vi "PhaSER-2C.vi"() -> ()   [LabVIEW 2017]
uses:
  Analog_Channels.ctl
  state_enum.ctl
  <vilib>/Analysis/3filter.llb/Filter Passband Type.ctl
  <vilib>/Analysis/3filter.llb/Filter Structure Type.ctl
  <vilib>/Utility/error.llb/DialogType.ctl
  <vilib>/DAQmx/read.llb/DAQmx Read (Analog 1D Wfm NChan NSamp).vi
  <vilib>/DAQmx/write.llb/DAQmx Write (Digital Bool 1Line 1Point).vi
  <vilib>/DAQmx/miscellaneous.llb/DAQmx Fill In Error Info.vi
  <vilib>/Analysis/3filter.llb/Zero Phase Filter (DBL).vi
  <vilib>/DAQmx/create/channels.llb/DAQmx Create Channel (AI-Voltage-Basic).vi
  <vilib>/DAQmx/configure/timing.llb/DAQmx Timing (Sample Clock).vi
  <vilib>/DAQmx/create/channels.llb/DAQmx Create Channel (DO-Digital Output).vi
  <vilib>/DAQmx/create/channels.llb/DAQmx Create Channel (CO-Pulse Generation-Time).vi
  <resource>/objmgr/daqmx.rc
  <vilib>/Analysis/NI_AALBase.lvlib
  <vilib>/ptbypt/NI_PtbyPt.lvlib
panel:
  in  "zero phase order":i32=1
  in  "low cutoff":dbl=4.0 format="%0.3f"
  in  "high cutoff":dbl=9.0 format="%0.3f"
  in  "Inhibition End":dbl=-45.0
  in  "Inhibtion Start":dbl=45.0
  in  "Inhibition Channel":tag="Dev1/PFI13"
  in  "timeout":dbl=100.0 caption="Pulse Timeout (ms)"
  in  "pulse phase":dbl format="%#_13g"
  in  "Counter":tag="Dev1/ctr0"
  in  "Output Terminal":tag="/Dev1/PFI12"
  in  "Pulse Duration":dbl=0.001 format="%.6f"
  out "Ball Tracker":i32=3
  out "Inhibition":i32=-1
  out "Pulse Train":i32=2
  out "Trigger":i32=1
  out "LFP":i32
  in  "Channel Assignments":T1[](array[typedef])=[enum."LFP", enum."Trigger", enum."Pulse Train", enum."Ball Tracker", enum."Inhibition"]
  in  "Samples to read":i32=25
  in  "Sample Rate":dbl=25000.0
  in  "Max Voltage":dbl=2.0
  in  "Min Voltage":dbl=-1.0
  in  "Physical Channel":tag="Dev1/ai0:4"
  in  "restrict to running?":bool=TRUE
  in  "fractional run threshold":dbl=0.1
  in  "lower speed bound":dbl=2.4 format="%#_13g"
  in  "upper speed bound":dbl=2.7 format="%#_13g"
  in  "sample length (ms)":i32=1000
  in  "Base Filename":path=path "C:/Users/Paul/Desktop/LabVIEW_Recordings/test"
  in  "Quit Button":bool
  in  "Stop Button":bool
  in  "Stimulate Button":bool
  in  "Baseline Button":bool
  in  "thickness":i32=150
  in  "width":i32=1000
  in  "p":dbl=13.0
  out "Waveform Chart":waveform(dbl)[](graph)=[{"t0"=timestamp(3702733252.213229 s since 1904-01-01), "dt"=0.001, "Y"=[-0.49778657094501827], "attributes"=variant("NI_ChannelName"=variant(string "Silicon Probe"), "NI_UnitDescription"=variant(string "Volts"))}, {"t0"=timestamp(3702733252.2132373 s since 1904-01-01), "dt"=3.9999999999999996e-05, "Y"=[0.0012770261409516398, 0.0009479371254728086, 0.0007833926177167883, 0.0009479371254728086, 0.0011124816332177545, 0.0009479371254728086, 0.0011124816332177545, 0.0009479371254728086, 0.0011124816332177545, 0.0009479371254728086, 0.0007833926177167883, 0.0007833926177167883, 0.0011124816332177545, 0.0011124816332177545, 0.0007833926177167883, 0.0011124816332177545, 0.0011124816332177545, 0.0007833926177167883, 0.0009479371254728086, 0.0009479371254728086, 0.0007833926177167883, 0.0011124816332177545, 0.0007833926177167883, 0.0011124816332177545, 0.0011124816332177545], "attributes"=variant("NI_ChannelName"=variant(string "Trigger"), "NI_UnitDescription"=variant(string "Volts"))}, {"t0"=timestamp(3702733252.2132454 s since 1904-01-01), "dt"=3.9999999999999996e-05, "Y"=[0.004897005308322218, 0.0045679162933244324, 0.004897005308322218, 0.0045679162933244324, 0.004732460800828724, 0.0045679162933244324, 0.004732460800828724, 0.004403371785809317, 0.004732460800828724, 0.0045679162933244324, 0.004732460800828724, 0.0045679162933244324, 0.004403371785809317, 0.004732460800828724, 0.004732460800828724, 0.0045679162933244324, 0.004403371785809317, 0.004732460800828724, 0.004732460800828724, 0.004403371785809317, 0.004732460800828724, 0.004732460800828724, 0.004403371785809317, 0.0045679162933244324, 0.005390638830738002], "attributes"=variant("NI_ChannelName"=variant(string "Pulse Train"), "NI_UnitDescription"=variant(string "Volts"))}, {"t0"=timestamp(3702733252.213253 s since 1904-01-01), "dt"=3.9999999999999996e-05, "Y"=[2.6063520142436025, 2.603883827309811, 2.6040483731041806, 2.608162018019915, 2.60668110583773, 2.5999347282970344, 2.604212918898724, 2.6052001936696327, 2.6117820256357307, 2.607174743230226, 2.607503834826093, 2.609972021817286, 2.6010865488321, 2.607174743230226, 2.5948338088867064, 2.602402915168302, 2.605858376853715, 2.604212918898724, 2.5890747065265556, 2.609478384415914, 2.607503834826093, 2.6043774646934414, 2.6027320067540884, 2.6043774646934414, 2.604542010488332], "attributes"=variant("NI_ChannelName"=variant(string "Ball Tracker"), "NI_UnitDescription"=variant(string "Volts"))}, {"t0"=timestamp(3702733252.213261 s since 1904-01-01), "dt"=3.9999999999999996e-05, "Y"=[2.562418292635671, 2.561924655383818, 2.5632410213921757, 2.5632410213921757, 2.5632410213921757, 2.563899204400454, 2.5637346586481278, 2.5637346586481278, 2.564063750152951, 2.5637346586481278, 2.563570112895973, 2.5625828383866303, 2.561760109633542, 2.562089201134265, 2.561266472383738, 2.562089201134265, 2.5622537468848825, 2.562089201134265, 2.562089201134265, 2.5622537468848825, 2.5622537468848825, 2.562418292635671, 2.562418292635671, 2.562089201134265, 2.5634055671439886], "attributes"=variant("NI_ChannelName"=variant(string "Inhibition"), "NI_UnitDescription"=variant(string "Volts"))}, {"t0"=timestamp(3702733252.213229 s since 1904-01-01), "dt"=0.001, "Y"=[0.32829558433683736], "attributes"=variant("NI_ChannelName"=variant(string "Predicted Signal"), "NI_UnitDescription"=variant(string "Volts"))}]
  out "Status":string="Quitting Program"
  # "Filter Parameters"
  # "Excitation Trigger"
  # "Inhibition TTL"
  # "Analog In Channels"
  # "Channel Number:"
  # "Analog In 0"
  # "Analog In 1"
  # "Analog In 2"
  # "Analog In 3"
  # "Analog In 4"
  # "Ball Tracker Parameters"
  # "Autoregression Parameters"
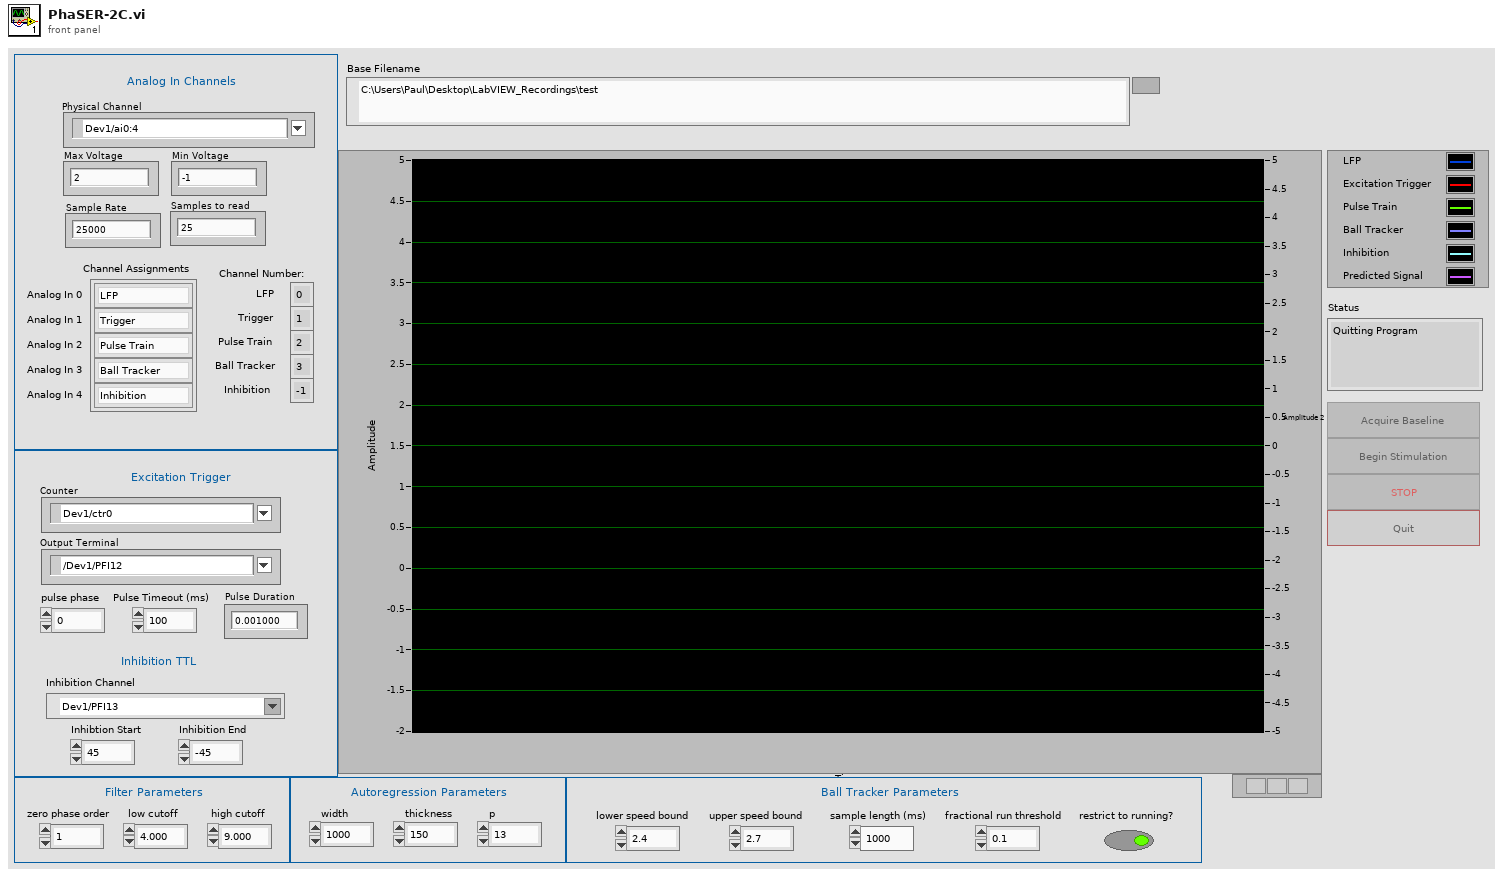
[diagram p1: front panel]
types:
  T1 = typedef "Analog_Channels.ctl" = enum16{"LFP", "Trigger", "Pulse Train", "Glass Electrode", "Ball Tracker", "Inhibition"}
  T2 = typedef "DialogType.ctl" = u16
  T3 = typedef "NI_AALBase.lvlib/Filter Structure Type.ctl" = u16
  T4 = typedef "NI_AALBase.lvlib/Filter Passband Type.ctl" = enum32{"Lowpass", "Highpass", "Bandpass", "Bandstop"}
  T5 = typedef "state_enum.ctl" = enum16{"Wait", "Locate", "Stop", "Quit", "Baseline", "Artifact", "Stimulate", "Initialize"}
  T6 = cluster{"filter structure":enum32{"IIR 2nd Order", "IIR 4th Order"}, "Reverse Coefficients":dbl[], "Forward Coefficients":dbl[]}
  T7 = enum16{"open", "open or create", "create or replace", "create", "open (read-only)"}
  T8 = enum8{"Enabled", "Disabled", "Disabled and Grayed Out"}
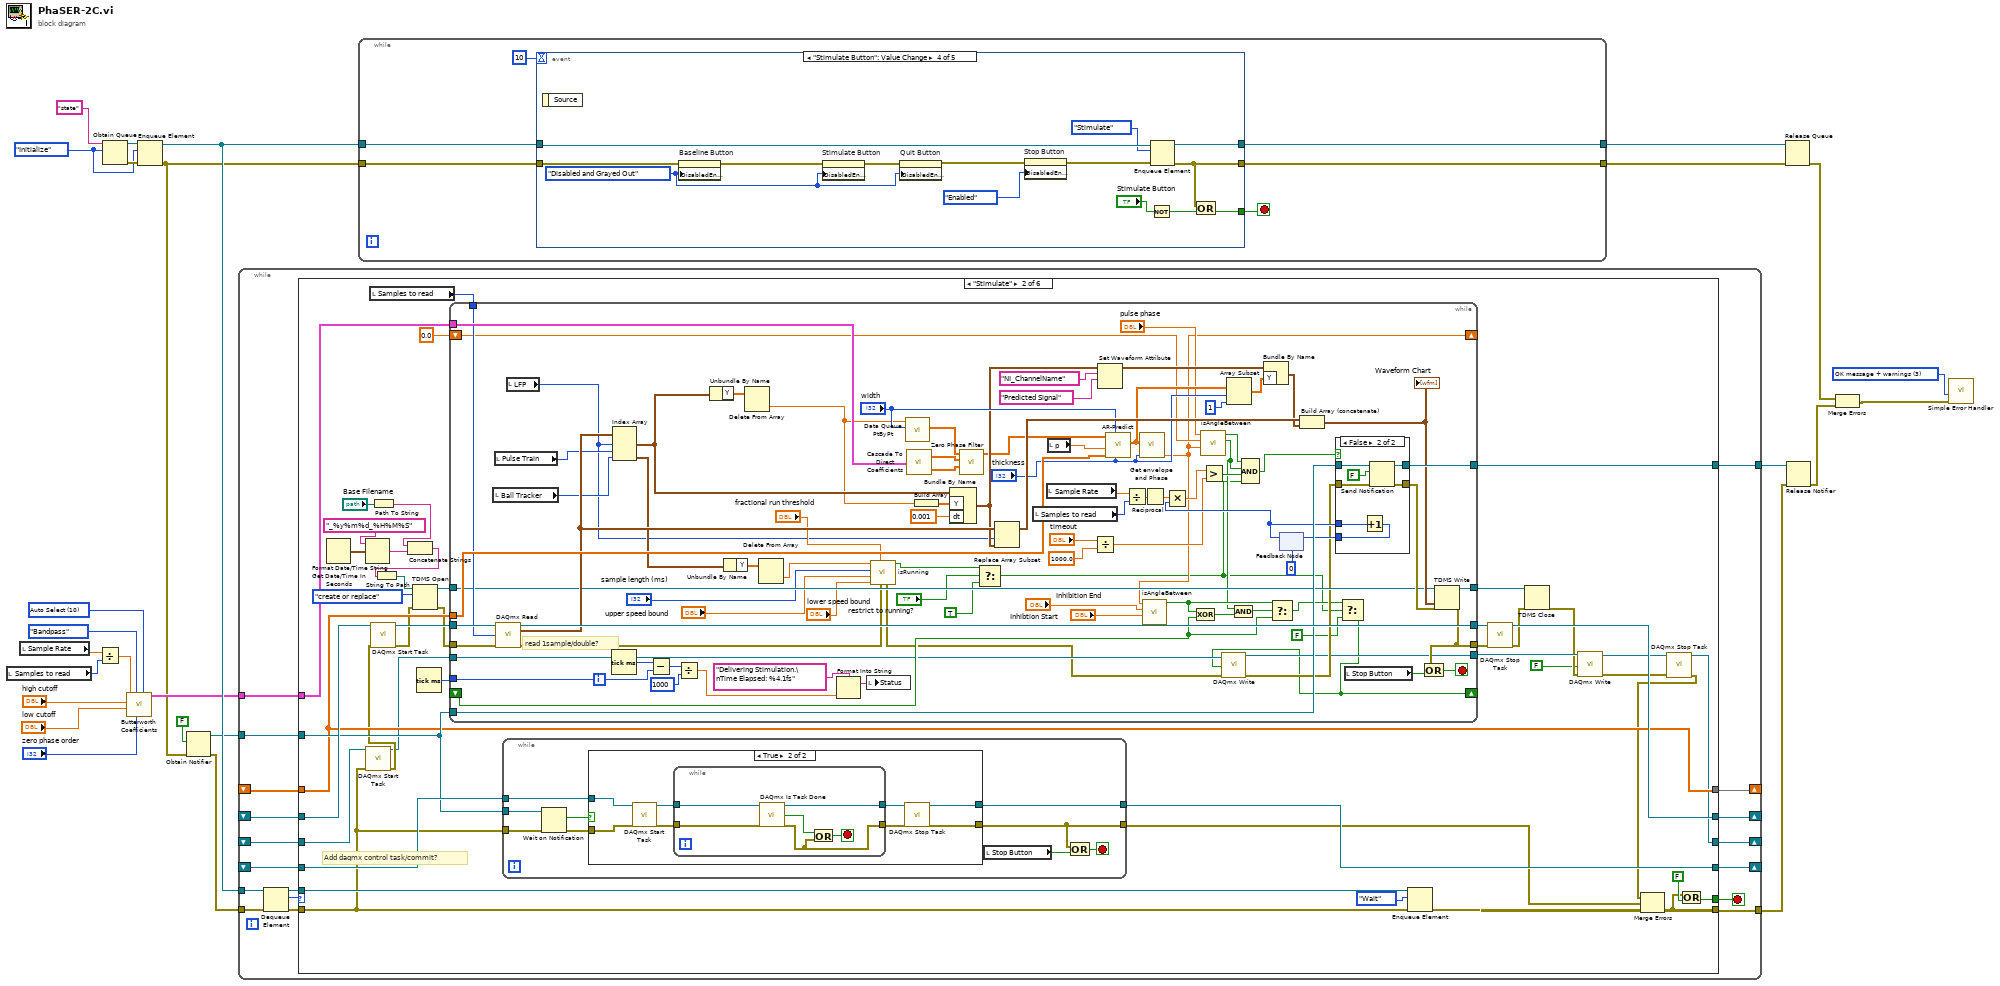
[diagram p0: block diagram]
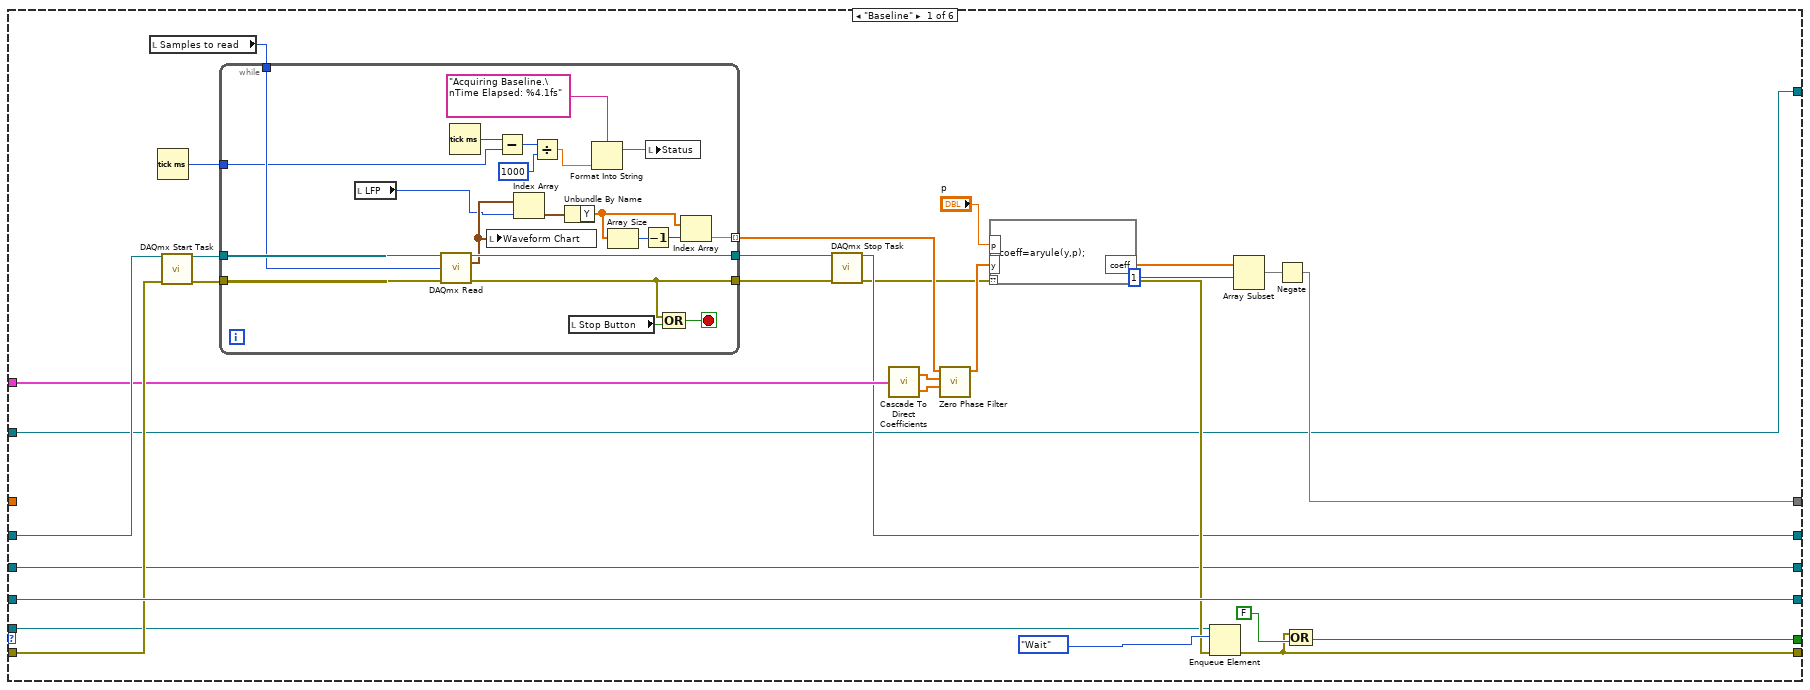
[diagram p2: hidden frame]
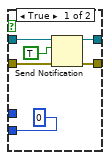
[diagram p4: hidden frame]
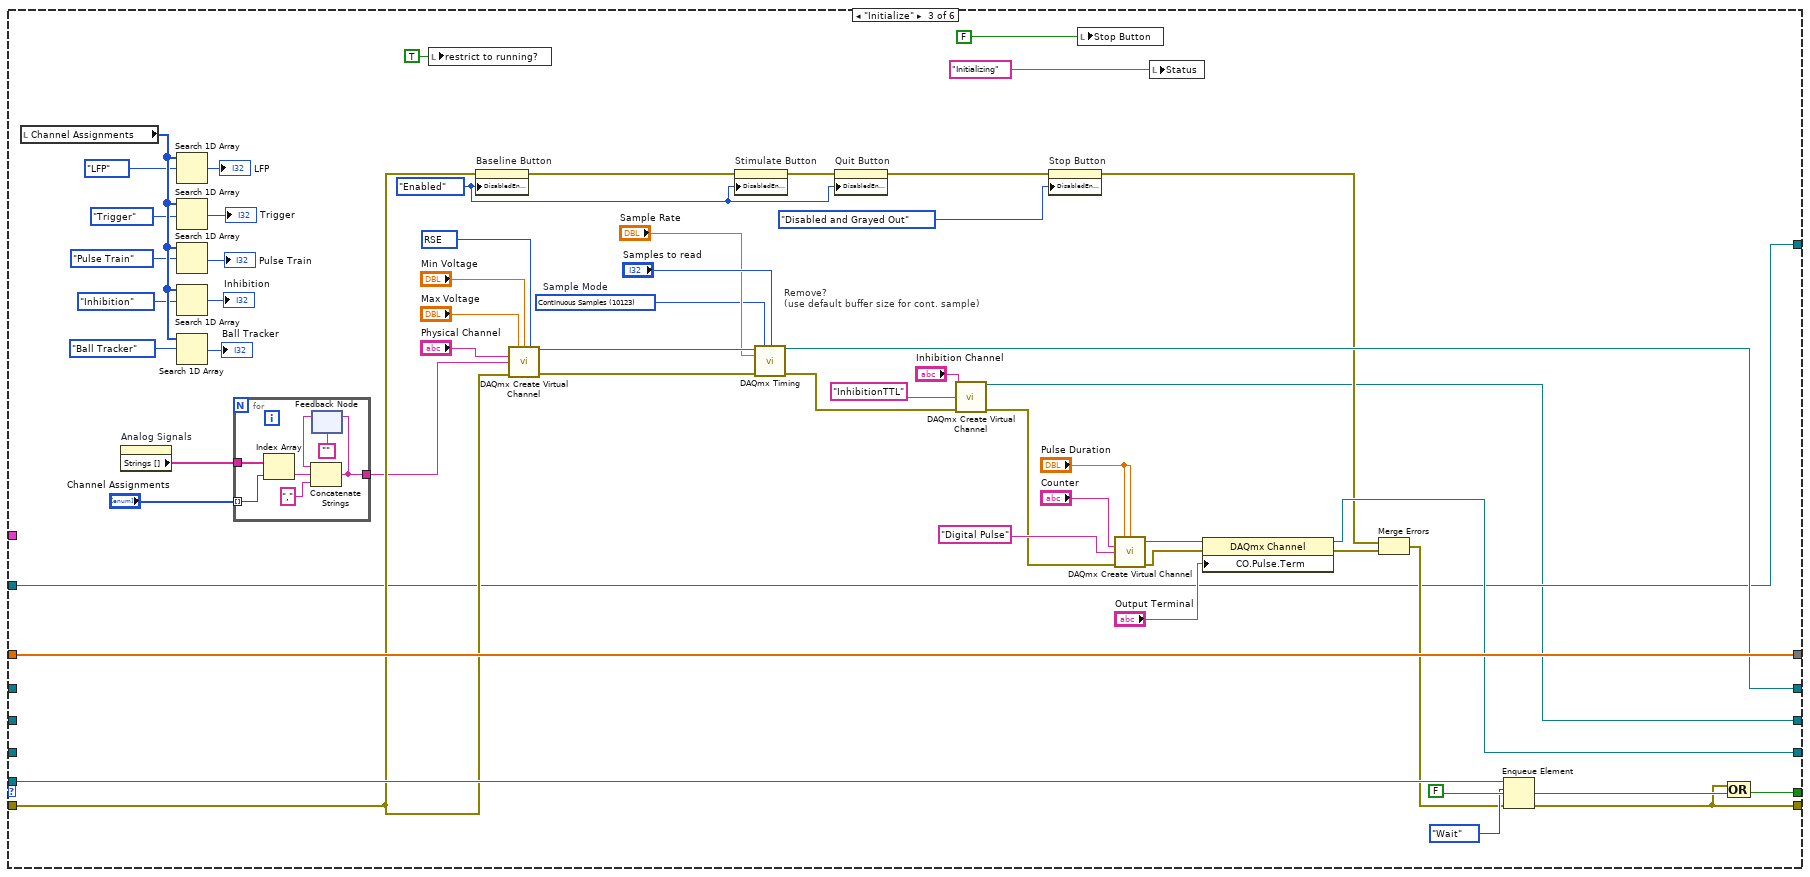
[diagram p5: hidden frame]
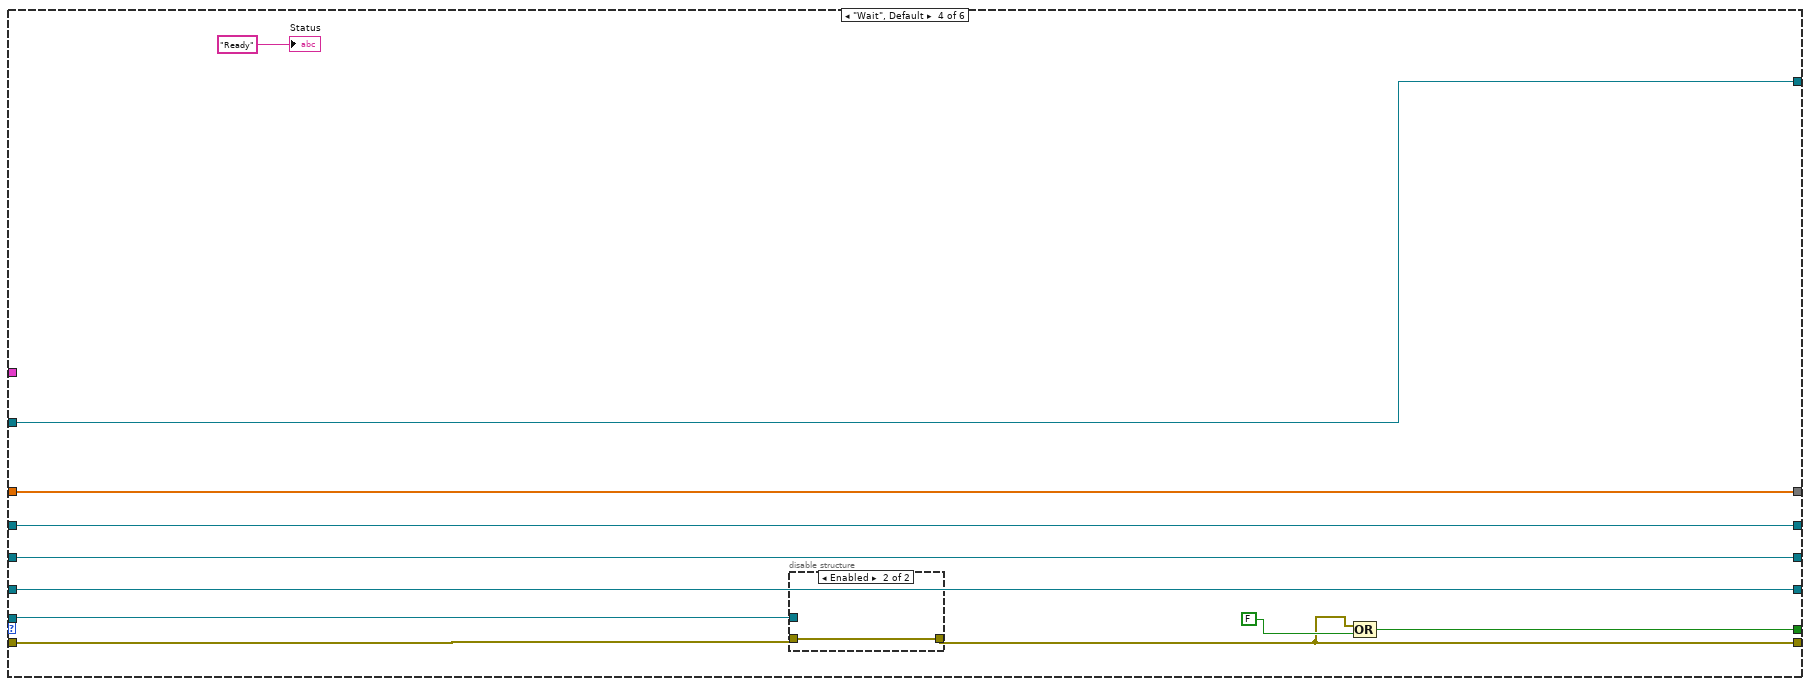
[diagram p6: hidden frame]
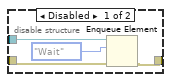
[diagram p7: hidden frame]
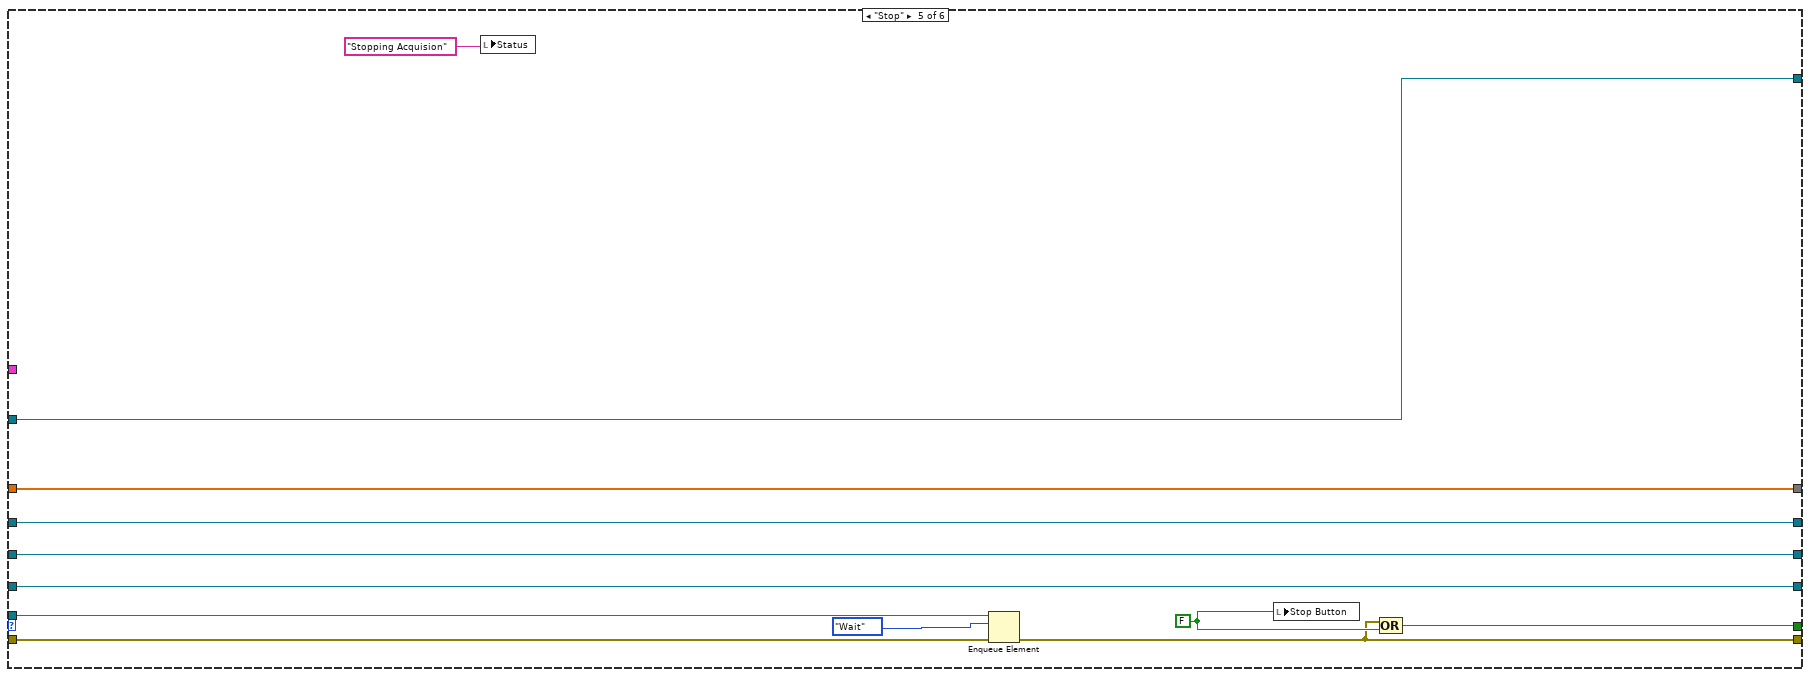
[diagram p8: hidden frame]
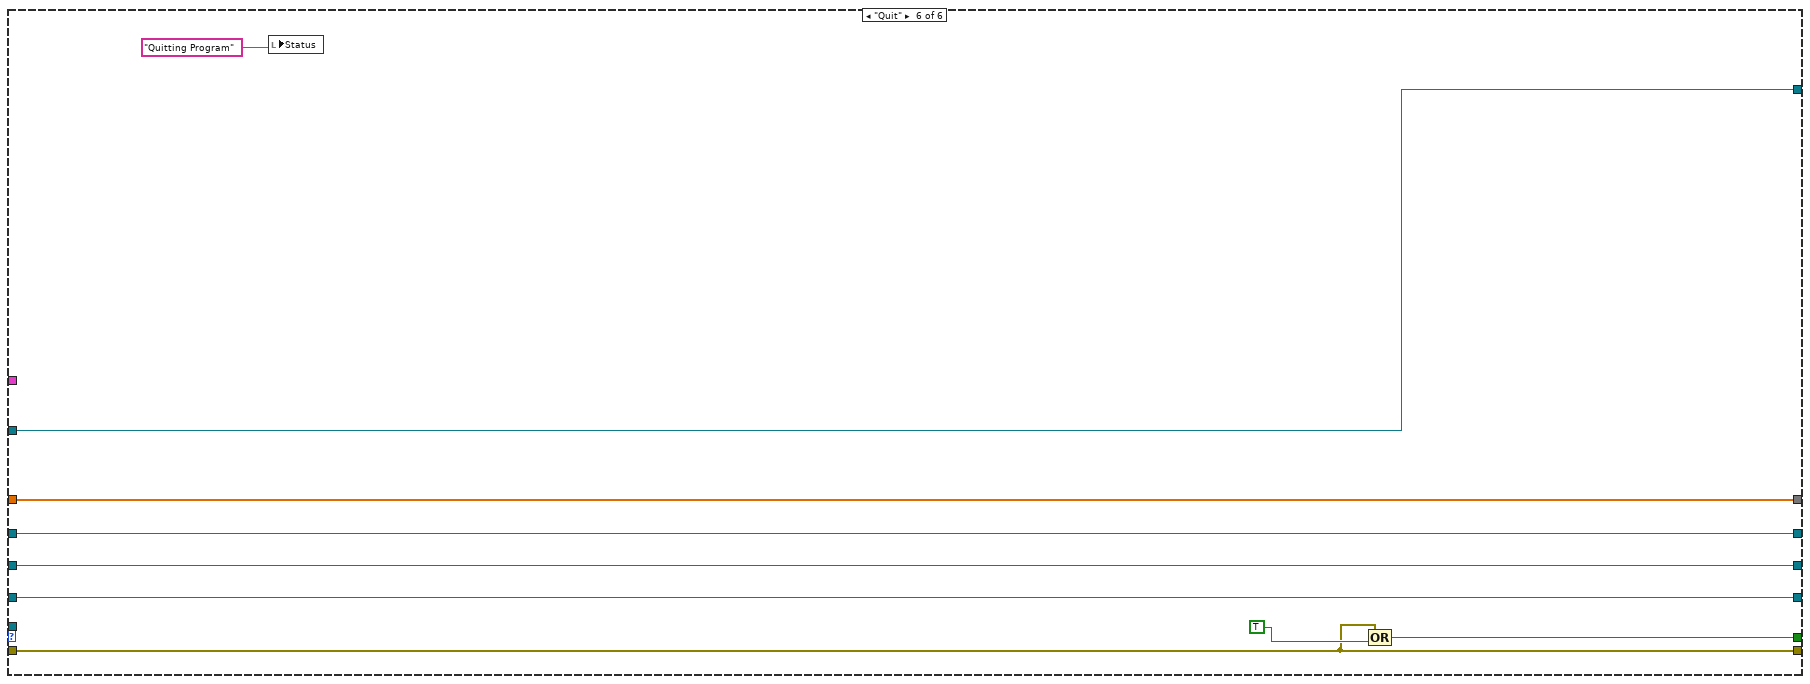
[diagram p9: hidden frame]
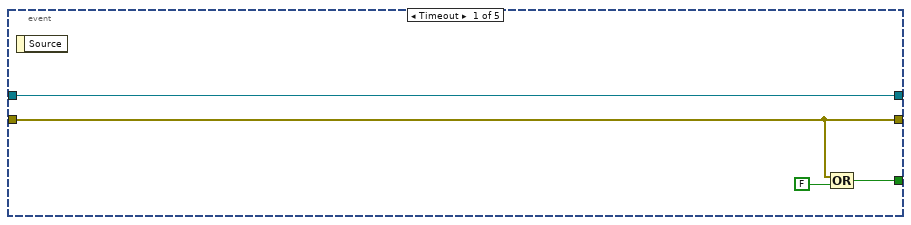
[diagram p10: hidden frame]
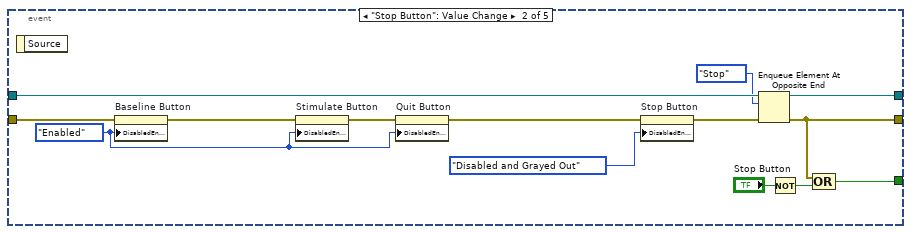
[diagram p11: hidden frame]
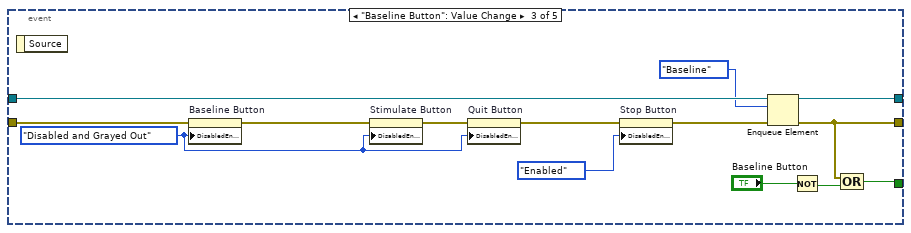
[diagram p12: hidden frame]
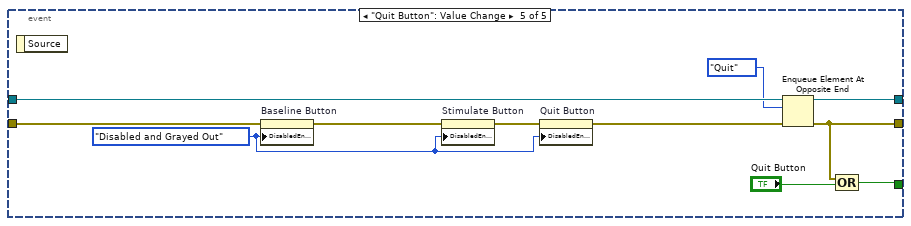
[diagram p13: hidden frame]
diagram:
  w9 = T2 3 items=["no dialog", "OK message", "continue or stop message", "OK message + warnings", "continue/stop + warnings"] ("type of dialog (OK msg:1)")
  w17 = T3 10 items=["IIR 2nd Order"=0, "IIR 4th Order"=1, "Auto Select"=10] ("filter structure option")
  w23 = state_enum."Initialize"
  n1 = local read "Samples to read"() -> (w4:i32)
  n2 = local read "Sample Rate"() -> (w14:dbl)
  n3 = Divide(x=w14, y=w4) -> (x/y=w1:dbl)
  n4 = Obtain Queue(name (unnamed)="state", element data type=w23) -> (queue out=w25:refnum<queue>, error out=w24:errorcluster)  [unwired: 3 in, 1 out]
  n5 = call <vilib>:"Butterworth Coefficients.vi"("filter structure option"=w17, "order"="zero phase order", "filter type"=Filter_Passband_Type."Bandpass", "low cutoff freq: fl"="low cutoff", "high cutoff freq: fh"="high cutoff", "sampling freq: fs"=w1) -> ("IIR Filter Cluster"=w15:T6)  [unwired: 4 in, 1 out]
  n6 = Enqueue Element(queue=w25, element=w23, error in (no error)=w24) -> (queue out=w22:refnum<queue>, error out=w11:errorcluster)  [unwired: 1 in, 1 out]
  n7 = Obtain Notifier(notification data type=FALSE, error in (no error)=w11) -> (notifier out=w12:refnum<notifier>, error out=w10:errorcluster)  [unwired: 1 in, 2 out]
  n8 = while {
    tunnel: w22 -> [w44]
    tunnel: [w41] -> w6
    shift-right: [w39] -> _
    shift-left: _ -> [w37]
    shift-right: [w38] -> _
    shift-left: _ -> [w36]
    tunnel: w15 -> [w34]
    shift-right: [w33] -> _
    shift-left: _ -> [w32]
    tunnel: w12 -> [w31]
    tunnel: w10 -> [w30]
    tunnel: [w29] -> w7
    shift-right: [w28] -> _
    shift-left: _ -> [w27]
    stop <- w40 stop-if-true
    n9 = Dequeue Element(queue=w44, error in (no error)=w30) -> (queue out=w35:refnum<queue>, element=w43:T5, error out=w42:errorcluster)  [unwired: 1 in, 1 out]
    n10 = case shown="\"Stimulate\"" w43 {
      tunnel: [w55 w121 w298 w331 w348 w364] -> w41
      tunnel: w42 -> [w69 w105 w295 w333 w352 w364]
      tunnel: [w72 w138 w321 w339 w349 w365] -> w40
      tunnel: [w49 w129 w300 w338 w357 w363] -> w39
      tunnel: [w71 w123 w301 w337 w356 w362] -> w38
      tunnel: w37 -> [w70 w137 _ w338 w357 w363]
      tunnel: w36 -> [w71 w125 _ w337 w356 w362]
      tunnel: w35 -> [w53 w133 w319 w332 w351 _]
      tunnel: w34 -> [w64 w127 _ _ _ _]
      tunnel: [w57 w122 w318 w336 w355 w361] -> w33
      tunnel: w32 -> [_ w122 w318 w336 w355 w361]
      tunnel: w31 -> [w46 w124 w291 w334 w347 w359]
      tunnel: [w46 w119 w291 w334 w347 w359] -> w29
      tunnel: [w45 w100 w272 w330 w346 w358] -> w28
      tunnel: w27 -> [w45 w104 _ w330 w346 w358]
      frame "Baseline" {
        n11 = local read "Samples to read"() -> (w52:i32)
        n12 = Tick Count (ms)() -> (millisecond timer value=w47:u32)
        n13 = call <vilib>:"DAQmx Start Task.vi"("task/channels in"=w70, "error in"=w69) -> ("task out"=w68:refnum<k21>, "error out"=w67:errorcluster)  [unwired: 12 in]
        n14 = while {
          tunnel: [w88] -> w63 mode=indexing
          tunnel: w68 -> [w87]
          tunnel: w67 -> [w86]
          tunnel: [w85] -> w50
          tunnel: [w84] -> w51
          tunnel: w52 -> [w83]
          tunnel: w47 -> [w81]
          stop <- w93 stop-if-true
          n15 = local read "LFP"() -> (w74:i32)
          n16 = call-poly <vilib>:"DAQmx Read.vi"("task/channels in"=w87, "number of samples per channel"=w83, "error in"=w86) -> ("task out"=w85:refnum<k21>, "data"=w75:waveform(dbl)[], "error out"=w84:errorcluster)  [unwired: 10 in]
          n17 = Tick Count (ms)() -> (millisecond timer value=w82:u32)
          n18 = local write "Waveform Chart"(w75) -> ()
          n19 = Subtract(x=w82, y=w81) -> (x-y=w80:u32)
          n20 = Index Array(array=w75, index=w74) -> (element=w92:waveform(dbl))
          n21 = Divide(x=w80, y=u32 1000) -> (x/y=w78:dbl)
          n22 = Unbundle By Name(w92) -> ("Y"=w89:dbl[])
          n23 = local read "Stop Button"() -> (w94:bool)
          n24 = Format Into String(format string="Acquiring Baseline.\nTime Elapsed: %4.1fs", w78) -> (resulting string=w76:string)  [unwired: 2 in, 1 out]
          n25 = Array Size(array=w89) -> (size(s)=w91:i32)
          n26 = Decrement(x=w91) -> (x-1=w90:i32)
          n27 = local write "Status"(w76) -> ()
          n28 = Compound Arithmetic op=OR(w84, w94) -> (w93:bool)
          n29 = Index Array(array=w89, index=w90) -> (element=w88:dbl)
        }
        n30 = call <vilib>:"DAQmx Stop Task.vi"("task/channels in"=w50, "error in"=w51) -> ("task out"=w49:refnum<k21>, "error out"=w48:errorcluster)  [unwired: 12 in]
        n31 = call <vilib>:"Cascade To Direct Coefficients.vi"("IIR Filter Cluster"=w64) -> ("Reverse Coefficients"=w65:dbl[], "Forward Coefficients"=w66:dbl[])
        n32 = call-poly <vilib>:"Zero Phase Filter.vi"("Forward Coefficients"=w66, "Reverse Coefficients"=w65, "X"=w63) -> ("Filtered X"=w62:dbl[])  [unwired: 7 in, 1 out]
        n33 = script code="coeff=aryule(y,p);"("??"=w48, "p"="p", "y"=w62) -> ("??"=w54:errorcluster, "coeff"=w58:dbl[])
        n34 = Enqueue Element(queue=w53, element=state_enum."Wait", error in (no error)=w54) -> (error out=w55:errorcluster)  [unwired: 1 in, 2 out]
        n35 = Array Subset(array=w58, index=1) -> (w60:dbl[])  [unwired: 1 in]
        n36 = Negate(x=w60) -> (-x=w57:dbl[])
        n37 = Compound Arithmetic op=OR(w55, FALSE) -> (w72:bool)
      }
      frame "Stimulate" {
        # "Add daqmx control task/commit?"
        n38 = Get Date/Time In Seconds() -> (seconds since 1Jan1904=w112:timestamp)
        n39 = Format Date/Time String(time format string (%c)="_%y%m%d_%H%M%S", seconds (now)=w112) -> (date/time string=w109:string)  [unwired: 1 in]
        n40 = call <vilib>:"DAQmx Start Task.vi"("task/channels in"=w104, "error in"=w105) -> ("task out"=w102:refnum<k21>, "error out"=w103:errorcluster)  [unwired: 12 in]
        n41 = local read "Samples to read"() -> (w132:i32)
        n42 = call <vilib>:"DAQmx Start Task.vi"("task/channels in"=w137, "error in"=w103) -> ("task out"=w136:refnum<k21>, "error out"=w117:errorcluster)  [unwired: 12 in]
        n43 = Path To String(path="Base Filename") -> (string=w108:string)
        n44 = Concatenate Strings(w108, w109) -> (w106:string)
        n45 = String To Path(string=w106) -> (path=w107:path)
        n46 = TDMS Open(8:w117, 10:T7."create or replace" ("operation (0:open)"), 11:w107) -> (0:w116:errorcluster, 3:w115:refnum<k34>)  [unwired: 4 in]
        n47 = Tick Count (ms)() -> (millisecond timer value=w128:u32)
        n48 = while {
          tunnel: w136 -> [w252]
          tunnel: w116 -> [w251]
          tunnel: [w250] -> w130
          tunnel: [w199] -> w131
          tunnel: w132 -> [w226]
          tunnel: w128 -> [w249]
          tunnel: w127 -> [w240]
          tunnel: w122 -> [w235]
          shift-right: [w176] -> _
          shift-left: 0.0 -> [w184]
          tunnel: w124 -> [w238]
          tunnel: [w237] -> w119
          tunnel: w115 -> [w200]
          tunnel: [w198] -> w114
          tunnel: w102 -> [w174]
          shift-right: [w167] -> _
          shift-left: _ -> [w175]
          tunnel: [w171] -> w99
          stop <- w253 stop-if-true
          # "read 1sample/double?"
          n49 = local read "Ball Tracker"() -> (w197:i32)
          n50 = local read "Pulse Train"() -> (w206:i32)
          n51 = call-poly <vilib>:"DAQmx Read.vi"("task/channels in"=w252, "number of samples per channel"=w226, "error in"=w251) -> ("task out"=w250:refnum<k21>, "data"=w232:waveform(dbl)[], "error out"=w190:errorcluster)  [unwired: 10 in]
          n52 = local read "LFP"() -> (w166:i32)
          n53 = Tick Count (ms)() -> (millisecond timer value=w234:u32)
          n54 = Index Array(array=w232, index #1=w166, index #2=w206, index #3=w197) -> (element #1=w233:waveform(dbl), element #3=w195:waveform(dbl))  [unwired: 1 out]
          n55 = Subtract(x=w234, y=w249) -> (x-y=w248:u32)
          n56 = Divide(x=w248, y=u32 1000) -> (x/y=w246:dbl)
          n57 = Unbundle By Name(w233) -> ("Y"=w165:dbl[])
          n58 = Unbundle By Name(w195) -> ("Y"=w196:dbl[])
          n59 = Delete From Array(array=w165) -> (deleted portion=w219:dbl)  [unwired: 2 in, 1 out]
          n60 = Delete From Array(array=w196) -> (deleted portion=w194:dbl)  [unwired: 2 in, 1 out]
          n61 = Format Into String(format string="Delivering Stimulation.\nTime Elapsed: %4.1fs", w246) -> (resulting string=w244:string)  [unwired: 2 in, 1 out]
          n62 = local write "Status"(w244) -> ()
          n63 = call "isRunning.vi"("error in (no error)"=w190, "fractional run \nthreshold"="fractional run threshold", "lower\nspeed bound"="lower speed bound", "upper\nspeed bound"="upper speed bound", "sample\nlength (ms)"="sample length (ms)", "ballspeed"=w194) -> ("isRunning?"=w188:bool, "error out"=w173:errorcluster)  [unwired: 4 in]
          n64 = call <vilib>:"Data Queue PtByPt.vi"("sample length"="width", "input data point"=w219) -> ("Current Queue"=w241:dbl[])  [unwired: 5 in, 4 out]
          n65 = call <vilib>:"Cascade To Direct Coefficients.vi"("IIR Filter Cluster"=w240) -> ("Reverse Coefficients"=w243:dbl[], "Forward Coefficients"=w242:dbl[])
          n66 = Build Array(w219) -> (w220:dbl[])
          n67 = Bundle By Name(cluster=w233, "Y"=w220, "dt"=0.001) -> (w228:waveform(dbl))
          n68 = call-poly <vilib>:"Zero Phase Filter.vi"("Forward Coefficients"=w242, "Reverse Coefficients"=w243, "X"=w241) -> ("Filtered X"=w224:dbl[])  [unwired: 7 in, 1 out]
          n69 = Select(t=w188, s="restrict to running?", f=TRUE) -> (s? t:f=w168:bool)
          n70 = Replace Array Subset(array=w232, new element=w228, index=w166) -> (w231:waveform(dbl)[])
          n71 = local read "Samples to read"() -> (w213:i32)
          n72 = local read "Sample Rate"() -> (w212:dbl)
          n73 = local read "p"() -> (w236:dbl)
          n74 = Divide(x="timeout", y=1000.0) -> (x/y=w207:dbl)
          n75 = Set Waveform Attribute(5:"Predicted Signal", 6:"NI_ChannelName", 7:w228) -> (3:w205:waveform(dbl))  [unwired: 1 in, 2 out]
          n76 = call "AR-Predict.vi"("thickness"="thickness", "width"="width", "AR coeff"=w235, "p"=w236, "filtered signal"=w224) -> ("predicted signal"=w223:dbl[])  [unwired: 6 in]
          n77 = Divide(x=w212, y=w213) -> (x/y=w211:dbl)
          n78 = call "Get envelope and Phase.vi"("thickness"="thickness", "signal"=w223) -> ("phase"=w176:dbl)  [unwired: 8 in, 1 out]
          n79 = call "isAngleBetween.vi"("End"="Inhibition End", "Start"="Inhibtion Start", "Angle"=w176) -> ("Between?"=w180:bool)  [unwired: 7 in, 1 out]
          n80 = Reciprocal(x=w211) -> (1/x=w210:dbl)
          n81 = Exclusive Or(1:w175, 2:w180) -> (0:w179:bool)
          n82 = call "isAngleBetween.vi"("End"=w176, "Start"=w184, "Angle"="pulse phase") -> ("Clockwise?"=w177:bool, "Between?"=w183:bool)  [unwired: 7 in]
          n83 = Array Subset(array=w223, index="thickness", length=1) -> (w229:dbl[])
          n84 = And(x=w177, y=w179) -> (x .and. y?=w178:bool)
          n85 = Bundle By Name(cluster=w205, "Y"=w229) -> (w227:waveform(dbl))
          n86 = Select(t=w180, s=w178, f=w175) -> (s? t:f=w170:bool)
          n87 = feedback #1(0) -> (w214:i32)
          n88 = Multiply(x=w210, y=w214) -> (x*y=w208:dbl)
          n89 = Greater?(x=w208, y=w207) -> (0:w209:bool)
          n90 = Compound Arithmetic op=AND(w183, w177, w209, w168) -> (w239:bool)
          n91 = Build Array (concatenate)(w231, w227) -> (w202:waveform(dbl)[])
          "Waveform Chart" <- w202
          n92 = Select(t=w170, s=w168, f=FALSE) -> (s? t:f=w167:bool)
          n93 = call-poly <vilib>:"DAQmx Write.vi"("task/channels in"=w174, "data"=w167, "error in"=w173) -> ("task out"=w171:refnum<k21>, "error out"=w172:errorcluster)  [unwired: 10 in, 1 out]
          n94 = case shown="False" w239 {
            tunnel: w172 -> [w260 w267]
            tunnel: [w259 w266] -> w201
            tunnel: [w258 w265] -> w237
            tunnel: w238 -> [w256 w263]
            tunnel: w214 -> [_ w262]
            tunnel: [0 w261] -> w215
            frame True {
              n95 = Send Notification(notification=TRUE, notifier=w256, error in (no error)=w260) -> (notifier out=w258:refnum<notifier>, error out=w259:errorcluster)
            }
            frame False {
              n96 = Increment(x=w262) -> (x+1=w261:i32)
              n97 = Send Notification(notification=FALSE, notifier=w263, error in (no error)=w267) -> (notifier out=w265:refnum<notifier>, error out=w266:errorcluster)
            }
          }
          n98 = feedback-in #1(w215) -> ()
          n99 = local read "Stop Button"() -> (w254:bool)
          n100 = TDMS Write(0:w200, 9:w202, 11:w201) -> (4:w198:refnum<k34>, 15:w199:errorcluster)  [unwired: 3 in, 2 out]
          n101 = Compound Arithmetic op=OR(w199, w254) -> (w253:bool)
        }
        n102 = while {
          tunnel: w125 -> [w148]
          tunnel: [w142] -> w120
          tunnel: [w147] -> w123
          tunnel: w124 -> [w146]
          tunnel: w105 -> [w145]
          stop <- w143 stop-if-true
          n103 = Wait on Notification(notifier=w146, error in (no error)=w145) -> (notification=w140:bool, error out=w141:errorcluster)  [unwired: 4 out]
          n104 = case shown="True" w140 {
            tunnel: w148 -> [w150 w154]
            tunnel: [w149 w153] -> w142
            tunnel: [w150 w152] -> w147
            tunnel: w141 -> [w149 w151]
            frame False {
            }
            frame True {
              n105 = call <vilib>:"DAQmx Start Task.vi"("task/channels in"=w154, "error in"=w151) -> ("task out"=w155:refnum<k21>, "error out"=w156:errorcluster)  [unwired: 12 in]
              n106 = while {
                tunnel: w155 -> [w164]
                tunnel: w156 -> [w163]
                tunnel: [w159] -> w158
                tunnel: [w161] -> w157
                stop <- w162 stop-if-true
                n107 = call <vilib>:"DAQmx Is Task Done.vi"("task/channels in"=w164, "error in"=w163) -> ("task out"=w161:refnum<k21>, "task done?"=w160:bool, "error out"=w159:errorcluster)  [unwired: 11 in]
                n108 = Compound Arithmetic op=OR(w160, w159) -> (w162:bool)
              }
              n109 = call <vilib>:"DAQmx Stop Task.vi"("task/channels in"=w157, "error in"=w158) -> ("task out"=w152:refnum<k21>, "error out"=w153:errorcluster)  [unwired: 12 in]
            }
          }
          n110 = local read "Stop Button"() -> (w144:bool)
          n111 = Compound Arithmetic op=OR(w142, w144) -> (w143:bool)
        }
        n112 = Enqueue Element(queue=w133, element=state_enum."Wait", error in (no error)=w105) -> (error out=w134:errorcluster)  [unwired: 1 in, 2 out]
        n113 = call <vilib>:"DAQmx Stop Task.vi"("task/channels in"=w130, "error in"=w131) -> ("task out"=w129:refnum<k21>, "error out"=w113:errorcluster)  [unwired: 12 in]
        n114 = TDMS Close(8:w113, 11:w114) -> (0:w98:errorcluster)  [unwired: 1 out]
        n115 = call-poly <vilib>:"DAQmx Write.vi"("task/channels in"=w99, "data"=FALSE, "error in"=w98) -> ("task out"=w96:refnum<k21>, "error out"=w97:errorcluster)  [unwired: 10 in, 1 out]
        n116 = call <vilib>:"DAQmx Stop Task.vi"("task/channels in"=w96, "error in"=w97) -> ("task out"=w100:refnum<k21>, "error out"=w101:errorcluster)  [unwired: 12 in]
        n117 = Merge Errors(w101, w120, w134) -> (w121:errorcluster)
        n118 = Compound Arithmetic op=OR(w121, FALSE) -> (w138:bool)
      }
      frame "Initialize" {
        w290 = T8."Enabled" ("Disabled")
        w304 = 10123 items=["Finite Samples"=10178, "Continuous Samples"=10123, "Hardware Timed Single Point"=12522]  # Sample Mode
        w303 = 10083 items=["default"=-1, "RSE"=10083, "NRSE"=10078, "Differential"=10106, "Pseudodifferential"=12529] ("Terminal Configuration")
        # "Remove?\n(use default buffer size for cont. sample)"
        n119 = local read "Channel Assignments"() -> (w282:T1[])
        n120 = property on="Analog Signals" class="Enum (strict)"() -> ("Strings []"=w269:string[])  [unwired: 2 in, 2 out]
        n121 = Search 1D Array(1D array=w282, element=Analog_Channels."LFP" ("Analog In 1")) -> (index of element=→"LFP":i32)  [unwired: 1 in]
        n122 = Search 1D Array(1D array=w282, element=Analog_Channels."Trigger" ("Analog In 1")) -> (index of element=→"Trigger":i32)  [unwired: 1 in]
        n123 = Search 1D Array(1D array=w282, element=Analog_Channels."Pulse Train" ("Analog In 1")) -> (index of element=→"Pulse Train":i32)  [unwired: 1 in]
        n124 = Search 1D Array(1D array=w282, element=Analog_Channels."Inhibition" ("Analog In 1")) -> (index of element=→"Inhibition":i32)  [unwired: 1 in]
        n125 = Search 1D Array(1D array=w282, element=Analog_Channels."Ball Tracker" ("Analog In 1")) -> (index of element=→"Ball Tracker":i32)  [unwired: 1 in]
        n126 = for {
          tunnel: w269 -> [w329]
          tunnel: "Channel Assignments" -> [w328] mode=indexing
          tunnel: [w324] -> w288
          n127 = Index Array(array=w329, index=w328) -> (element=w327:string)
          n128 = feedback #2("") -> (w326:string)
          n129 = Concatenate Strings(w326, w327, "," ("string")) -> (w324:string)
          n130 = feedback-in #2(w324) -> ()
        }
        n131 = local write "restrict to running?"(TRUE ("restrict to running?")) -> ()
        n132 = property on="Baseline Button" class="Bool"(error in=w295, "DisabledEnum"=w290) -> (error out=w271:errorcluster)  [unwired: 1 in, 1 out]
        n133 = call-poly <vilib>:"DAQmx Create Virtual Channel.vi"("maximum value"="Max Voltage", "minimum value"="Min Voltage", "input terminal configuration"=w303, "physical channels"="Physical Channel", "name to assign"=w288, "error in"=w295) -> ("task out"=w316:refnum<k21>, "error out"=w315:errorcluster)  [unwired: 8 in]
        n134 = property on="Stimulate Button" class="Bool"(error in=w271, "DisabledEnum"=w290) -> (error out=w296:errorcluster)  [unwired: 1 in, 1 out]
        n135 = call-poly <vilib>:"DAQmx Timing.vi"("task/channels in"=w316, "sample mode"=w304, "samples per channel"="Samples to read", "rate"="Sample Rate", "error in"=w315) -> ("task out"=w300:refnum<k21>, "error out"=w274:errorcluster)  [unwired: 9 in]
        n136 = property on="Quit Button" class="Bool"(error in=w296, "DisabledEnum"=w290) -> (error out=w270:errorcluster)  [unwired: 1 in, 1 out]
        n137 = call-poly <vilib>:"DAQmx Create Virtual Channel.vi"("lines"="Inhibition Channel", "name to assign"="InhibitionTTL", "error in"=w274) -> ("task out"=w272:refnum<k21>, "error out"=w273:errorcluster)  [unwired: 11 in]
        n138 = property on="Stop Button" class="Bool (strict)"(error in=w270, "DisabledEnum"=T8."Disabled and Grayed Out" ("Disabled")) -> (error out=w293:errorcluster)  [unwired: 1 in, 1 out]
        n139 = local write "Stop Button"(FALSE ("Stop Button")) -> ()
        n140 = call-poly <vilib>:"DAQmx Create Virtual Channel.vi"("high time"="Pulse Duration", "low time"="Pulse Duration", "counter"="Counter", "name to assign"="Digital Pulse", "error in"=w273) -> ("task out"=w309:refnum<k21>, "error out"=w308:errorcluster)  [unwired: 9 in]
        n141 = local write "Status"("Initializing") -> ()
        n142 = property class="DAQmx Channel"(reference=w309, error in=w308, "CO.Pulse.Term"="Output Terminal") -> (reference out=w301:refnum<k21>, error out=w302:errorcluster)
        n143 = Merge Errors(w293, w302) -> (w294:errorcluster)
        n144 = Enqueue Element(queue=w319, element=state_enum."Wait", error in (no error)=w294) -> (error out=w298:errorcluster)  [unwired: 1 in, 2 out]
        n145 = Compound Arithmetic op=OR(w298, FALSE) -> (w321:bool)
      }
      frame "Wait", Default {
        n146 = disable-structure shown="Enabled" {
          disable-tunnel: w333 -> [w344 w345]
          disable-tunnel: w332 -> [w343 _]
          disable-tunnel: [w341 w345] -> w331
          frame Disabled {
            n147 = Enqueue Element(queue=w343, element=state_enum."Wait", error in (no error)=w344) -> (error out=w341:errorcluster)  [unwired: 1 in, 2 out]
          }
          frame Enabled {
          }
        }
        n148 = Compound Arithmetic op=OR(w331, FALSE) -> (w339:bool)
        "Status" <- "Ready"
      }
      frame "Stop" {
        w354 = FALSE
        n149 = local write "Status"("Stopping Acquision") -> ()
        n150 = Enqueue Element(queue=w351, element=state_enum."Wait", error in (no error)=w352) -> (error out=w348:errorcluster)  [unwired: 1 in, 2 out]
        n151 = local write "Stop Button"(w354) -> ()
        n152 = Compound Arithmetic op=OR(w348, w354) -> (w349:bool)
      }
      frame "Quit" {
        n153 = local write "Status"("Quitting Program") -> ()
        n154 = Compound Arithmetic op=OR(w364, TRUE) -> (w365:bool)
      }
    }
  }
  n155 = while {
    tunnel: w22 -> [w370]
    tunnel: w11 -> [w369]
    tunnel: [w368] -> w21
    tunnel: [w367] -> w20
    stop <- w371 stop-if-true
    n156 = event shown="[3] \"Stimulate Button\": Value Change" {
      selector: _ -> [_ _ _ _ _]
      dyn-events: _ -> [_ _ _ _ _]
      timeout: 10 -> [_ _ _ _ _]
      tunnel: [w374 w384 w399 w414 w425] -> w371
      tunnel: w370 -> [w373 w389 w403 w416 w429]
      tunnel: w369 -> [w376 w381 w396 w410 w422]
      tunnel: [w376 w387 w400 w413 w426] -> w368
      tunnel: [w373 w385 w398 w412 w424] -> w367
      event Timeout {
        n157 = event-data() -> ()  [unwired: 1 in, 1 out]
        n158 = Compound Arithmetic op=OR(w376, FALSE) -> (w374:bool)
      }
      event "Stop Button": Value Change {
        w379 = T8."Enabled" ("Disabled")
        n159 = event-data() -> ()  [unwired: 1 in, 1 out]
        n160 = property on="Baseline Button" class="Bool"(error in=w381, "DisabledEnum"=w379) -> (error out=w378:errorcluster)  [unwired: 1 in, 1 out]
        n161 = property on="Stimulate Button" class="Bool"(error in=w378, "DisabledEnum"=w379) -> (error out=w383:errorcluster)  [unwired: 1 in, 1 out]
        n162 = property on="Quit Button" class="Bool"(error in=w383, "DisabledEnum"=w379) -> (error out=w377:errorcluster)  [unwired: 1 in, 1 out]
        n163 = property on="Stop Button" class="Bool (strict)"(error in=w377, "DisabledEnum"=T8."Disabled and Grayed Out" ("Disabled")) -> (error out=w380:errorcluster)  [unwired: 1 in, 1 out]
        n164 = Enqueue Element At Opposite End(queue=w389, element=state_enum."Stop", error in (no error)=w380) -> (queue out=w385:refnum<queue>, error out=w387:errorcluster)  [unwired: 1 in, 1 out]
        n165 = Not(x="Stop Button") -> (.not. x?=w386:bool)
        n166 = Compound Arithmetic op=OR(w387, w386) -> (w384:bool)
      }
      event "Baseline Button": Value Change {
        w391 = T8."Disabled and Grayed Out" ("Disabled")
        n167 = event-data() -> ()  [unwired: 1 in, 1 out]
        n168 = property on="Baseline Button" class="Bool"(error in=w396, "DisabledEnum"=w391) -> (error out=w392:errorcluster)  [unwired: 1 in, 1 out]
        n169 = property on="Stimulate Button" class="Bool"(error in=w392, "DisabledEnum"=w391) -> (error out=w397:errorcluster)  [unwired: 1 in, 1 out]
        n170 = property on="Quit Button" class="Bool"(error in=w397, "DisabledEnum"=w391) -> (error out=w393:errorcluster)  [unwired: 1 in, 1 out]
        n171 = property on="Stop Button" class="Bool (strict)"(error in=w393, "DisabledEnum"=T8."Enabled" ("Disabled")) -> (error out=w394:errorcluster)  [unwired: 1 in, 1 out]
        n172 = Enqueue Element(queue=w403, element=state_enum."Baseline", error in (no error)=w394) -> (queue out=w398:refnum<queue>, error out=w400:errorcluster)  [unwired: 1 in, 1 out]
        n173 = Not(x="Baseline Button") -> (.not. x?=w401:bool)
        n174 = Compound Arithmetic op=OR(w400, w401) -> (w399:bool)
      }
      event "Stimulate Button": Value Change {
        w407 = T8."Disabled and Grayed Out" ("Disabled")
        n175 = event-data() -> ()  [unwired: 1 in, 1 out]
        n176 = property on="Baseline Button" class="Bool"(error in=w410, "DisabledEnum"=w407) -> (error out=w405:errorcluster)  [unwired: 1 in, 1 out]
        n177 = property on="Stimulate Button" class="Bool"(error in=w405, "DisabledEnum"=w407) -> (error out=w411:errorcluster)  [unwired: 1 in, 1 out]
        n178 = property on="Quit Button" class="Bool"(error in=w411, "DisabledEnum"=w407) -> (error out=w406:errorcluster)  [unwired: 1 in, 1 out]
        n179 = property on="Stop Button" class="Bool (strict)"(error in=w406, "DisabledEnum"=T8."Enabled" ("Disabled")) -> (error out=w408:errorcluster)  [unwired: 1 in, 1 out]
        n180 = Not(x="Stimulate Button") -> (.not. x?=w417:bool)
        n181 = Enqueue Element(queue=w416, element=state_enum."Stimulate", error in (no error)=w408) -> (queue out=w412:refnum<queue>, error out=w413:errorcluster)  [unwired: 1 in, 1 out]
        n182 = Compound Arithmetic op=OR(w413, w417) -> (w414:bool)
      }
      event "Quit Button": Value Change {
        w421 = T8."Disabled and Grayed Out" ("Disabled")
        n183 = event-data() -> ()  [unwired: 1 in, 1 out]
        n184 = property on="Baseline Button" class="Bool"(error in=w422, "DisabledEnum"=w421) -> (error out=w420:errorcluster)  [unwired: 1 in, 1 out]
        n185 = property on="Stimulate Button" class="Bool"(error in=w420, "DisabledEnum"=w421) -> (error out=w423:errorcluster)  [unwired: 1 in, 1 out]
        n186 = property on="Quit Button" class="Bool"(error in=w423, "DisabledEnum"=w421) -> (error out=w419:errorcluster)  [unwired: 1 in, 1 out]
        n187 = Enqueue Element At Opposite End(queue=w429, element=state_enum."Quit", error in (no error)=w419) -> (queue out=w424:refnum<queue>, error out=w426:errorcluster)  [unwired: 1 in, 1 out]
        n188 = Compound Arithmetic op=OR(w426, "Quit Button") -> (w425:bool)
      }
    }
  }
  n189 = Release Queue(queue=w20, error in (no error)=w21) -> (error out=w19:errorcluster)  [unwired: 1 in, 2 out]
  n190 = Release Notifier(notifier=w7, error in (no error)=w6) -> (error out=w5:errorcluster)  [unwired: 3 out]
  n191 = Merge Errors(w19, w5) -> (w8:errorcluster)
  n192 = call <vilib>:"Simple Error Handler.vi"("type of dialog (OK msg:1)"=w9, "error in (no error)"=w8) -> ()  [unwired: 3 in, 5 out]
